vi "example_bricker_i2c.vi"() -> ()   [LabVIEW 2022 SP3]
uses:
  <vilib>/Instr/_visa.llb/VISA Configure Serial Port (Instr).vi
panel:
  in  "VISA resource name":refnum<visa-resource-name>
  in  "stop":bool
  out "PRESSURE_DATA":string[](array[string])
  out "TEMP_DATA":string[](array[string])
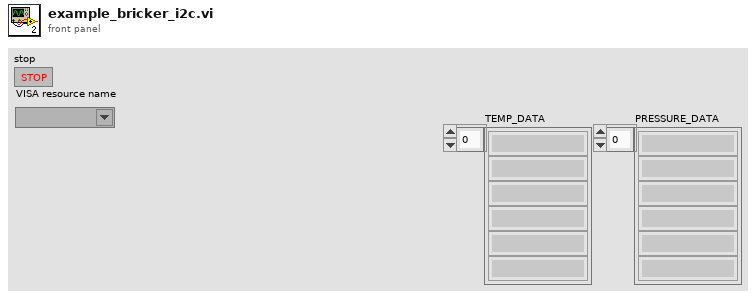
[diagram p1: front panel]
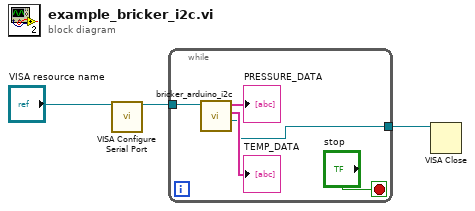
[diagram p0: block diagram]
diagram:
  n1 = call-poly "VISA Configure Serial Port"("VISA resource name"="VISA resource name") -> ("VISA resource name out"=w2:refnum<visa-resource-name>)  [unwired: 13 in, 1 out]
  n2 = while {
    tunnel: w2 -> [w5]
    tunnel: [w4] -> w1
    stop <- "stop" stop-if-true
    n3 = call "bricker_arduino_i2c.vi"("VISA resource name"=w5) -> ("VISA resource name out"=w4:refnum<visa-resource-name>, "TEMP_DATA"=→"TEMP_DATA":string[], "PRESSURE_DATA"=→"PRESSURE_DATA":string[])  [unwired: 8 in]
  }
  n4 = VISA Close(VISA resource name=w1) -> ()  [unwired: 1 in, 1 out]
